vi "Begin.vi"(8 "error in":errorcluster) -> (0 "error out":errorcluster)   [LabVIEW 2014]
doc: "Called before other user functions, this VI is expected to open initial I/O refnums, load in file data, and do all program initialization. Notice that the <B>error out</B> terminal is simply used for data flow. Wiring it to other structures or subVIs ensures that this VI runs first."
uses:
  Robot/Forward Drive/Forward Drive Class/Forward Drive Config.ctl
  Robot/Motor with Encoders/Motors with Encoders Class/Motors with Encoders.lvclass
  Robot Actor Framework/Trace/Trace Controller Class/Config.ctl
  Robot/Motor with Encoders/Motors with Encoders Class/Motors with Encoders Config.ctl
  Comp Robot/Comp Motors with Encoders/Comp Motors with Encoders Class/Motor Controller Config.ctl
  Comp Robot/Comp Motors with Encoders/Comp Motors with Encoders Class/Encoder Config.ctl
  Robot/Driver/Driver Class/Driver Config.ctl
  Robot/Joystick/Joystick Class/Joystick.lvclass
  <vilib>/ActorFramework/Message Enqueuer/Message Enqueuer.lvclass
  Robot/Sideways Drive/Sideways Drive Class/Sideways Drive Config.ctl
  Comp Robot/Comp Xbox One Controller/Comp XBox One Controller Class/Comp X1 Config.ctl
  <vilib>/Rock Robotics/WPI/Joystick/WPI_JoystickDeviceEnum.ctl
  Dev Grabber/Dev Grabber Class/Dev Grabber Config.ctl
  <vilib>/Rock Robotics/WPI/Solenoid/WPI_SolenoidChannel.ctl
  Robot/Operator/Operator Class/Operator Config.ctl
  Robot/Elevator/Elevator Class/Elevator Config.ctl
  Comp Robot/Comp Motors with Brake/Comp Motors with Brake Class/Comp Motors with Brake Config.ctl
  <vilib>/Rock Robotics/WPI/DriverStation/WPI_DriverStationRobotMode2.ctl
  Comp Robot/Comp Pressure/Comp Pressure Class/Comp Pressure.lvclass
  Robot/Forward Drive/Forward Drive Class/Forward Drive.lvclass
  Robot/Sideways Drive/Sideways Drive Class/Sideways Drive.lvclass
  Comp Robot/Comp Trace Controller/Comp Trace Controller Class/Comp Trace Controller.lvclass
  Comp Robot/Comp Xbox One Controller/Comp XBox One Controller Class/Comp XBox One Controller.lvclass
  Robot/Driver/Driver Class/Driver.lvclass
  Robot/Operator/Operator Class/Operator.lvclass
  Robot/Joystick/Joystick Class/Config.ctl
  Comp Robot/Comp Motors with Encoders/Comp Motors with Encoders Class/Comp Motors with Encoders.lvclass
  Dev Grabber/Dev Grabber Class/Dev Grabber.lvclass
  Comp Robot/Comp Motors with Brake/Comp Motors with Brake Class/Comp Motors with Brake.lvclass
  Robot/Elevator/Elevator Class/Elevator.lvclass
  Robot/Joystick/Joystick Class/Joystick.lvclass/Joystick.ctl
  Comp Robot/Comp Xbox One Controller/Comp XBox One Controller Class/Comp XBox One Controller.lvclass/Comp XBox One Controller.ctl
  Robot Global Data.vi
  <vilib>/ActorFramework/Actor/Actor.lvclass
  Robot Actor Framework/Trace/Trace Controller Class/Trace Controller.lvclass
panel:
  in  "Configs":T1(tab)=enum."Sideways Motors "
  in  "Trace Controller Config":T2={"Folder Pattern"="/media/sd%s1", "Starting Letter Position"=1, "Min Free Space (MB)"=50.0, "Max Folders to Check"=10, "Trace Level"=enum."Informational"} {"Min Free Space (MB)" format="%#_13g"}
  in  "Left Motors Config":T3={"Counts  Per Revolution"=256, "Invert Encoder Direction"=FALSE, "Diameter of Revolution"=6.0, "Max RPM"=1500.0, "Encoder Control"=TRUE}
  in  "Left Master Motor Controller Config":T4={"Device Number"=9, "Invert Motor"=FALSE}
  in  "Left Slave Motor Controller Configs":T4[](array[typedef])=[{"Device Number"=10, "Invert Motor"=FALSE}]
  in  "Left Encoder Config":T5={"P"=1.0, "D"=0.0, "F"=0.01, "I"=0.01, "Reverse Feedback Sensor"=TRUE, "Encoder Codes Per Rev"=256}
  in  "Right Encoder Config 2":T3={"Counts  Per Revolution"=256, "Invert Encoder Direction"=FALSE, "Diameter of Revolution"=6.0, "Max RPM"=1500.0, "Encoder Control"=TRUE}
  in  "Right Master Motor Controller Config":T4={"Device Number"=4, "Invert Motor"=TRUE}
  in  "Right Slave Motor Controller Configs":T4[](array[typedef])=[{"Device Number"=5, "Invert Motor"=FALSE}]
  in  "Right Encoder Config":T5={"P"=1.0, "D"=0.0, "F"=0.01, "I"=0.01, "Reverse Feedback Sensor"=TRUE, "Encoder Codes Per Rev"=256}
  in  "Forward Drive Config":T6={"Left Motors with Encoders"=refnum, "Right Motors with Encoders"=refnum, "Encoder Control"=TRUE}
  in  "Driver Config":T7={"Joystick"=refnum, "Forward Drive"=refnum, "Sideways Drive"=refnum, "Percent Forward"=1.0, "Percent Sideways"=1.0}
  in  "Driver X1 Config":T8={"Joystick USB"=enum."USB 0", "Deadband"=0.1}
  in  "Sideways - Motors with Encoder Config":T3={"Counts  Per Revolution"=256, "Invert Encoder Direction"=FALSE, "Diameter of Revolution"=6.0, "Max RPM"=1500.0, "Encoder Control"=TRUE}
  in  "Sideways Drive Config":T10
  in  "Sideways Encoder Config":T5={"P"=1.0, "D"=0.0, "F"=0.01, "I"=0.01, "Reverse Feedback Sensor"=FALSE, "Encoder Codes Per Rev"=256}
  in  "Sideways Master Motor Controller Config":T4={"Device Number"=11, "Invert Motor"=TRUE}
  in  "Sideways Slave Motor Controller Configs":T4[](array[typedef])=[{"Device Number"=6, "Invert Motor"=FALSE}]
  in  "Operator XBox One Controller Config":T8={"Joystick USB"=enum."USB 1", "Deadband"=0.1}
  in  "Operator Config":T11
  in  "Dev Grabber Config":T12={"PCM CAN ID"=3, "Forward Solenoid Channel"=enum."Solenoid 0", "Reverse Solenoid Channel"=enum."Solenoid 1", "Left Motor CAN ID"=13, "Right Motor CAN ID"=8, "Left Motor Invert"=FALSE, "Right Motor Invert"=TRUE}
  in  "Elevator Config":T14
  in  "Elevator Master Motor Controller Config":T4={"Device Number"=7, "Invert Motor"=FALSE}
  in  "Ellevator  Motor Controller Configs":T4[](array[typedef])
  in  "Elevator Encoder Config":T5={"P"=1.0, "D"=0.0, "F"=0.01, "I"=0.01, "Reverse Feedback Sensor"=FALSE, "Encoder Codes Per Rev"=256}
  in  "Elevator Motors with Encoders Config":T3={"Counts  Per Revolution"=256, "Invert Encoder Direction"=FALSE, "Diameter of Revolution"=1.5, "Max RPM"=1000.0, "Encoder Control"=TRUE}
  in  "Comp Motors with Brake Config":T15={"Brake Channel"=enum."Solenoid 6", "Pneumatics CAN ID"=3}
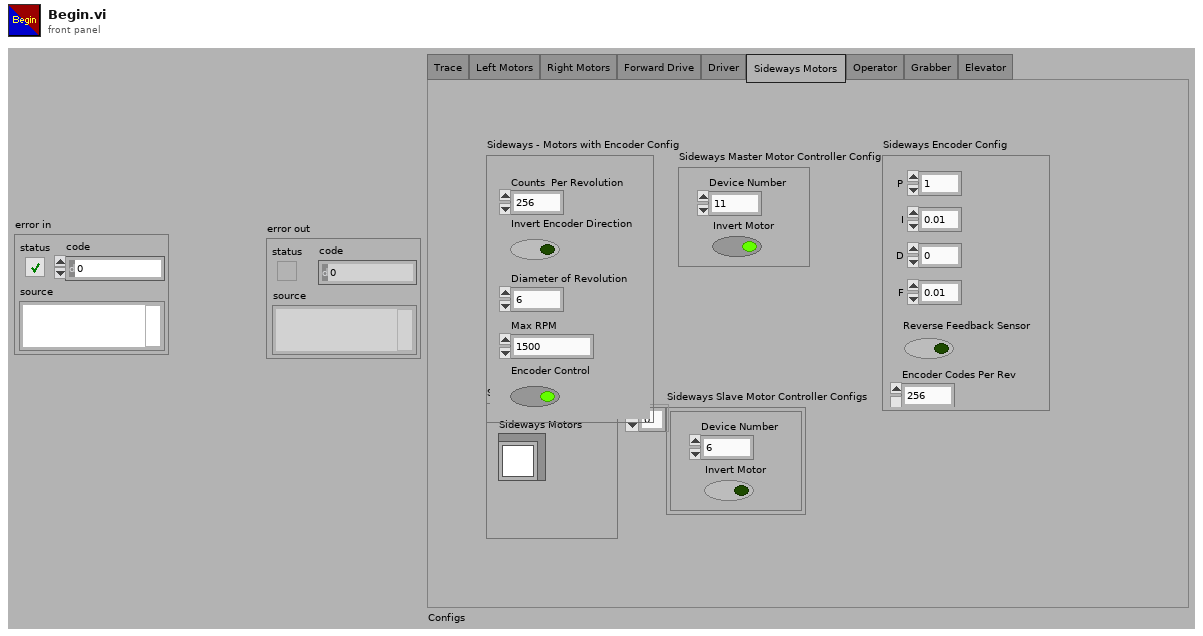
[diagram p1: front panel]
types:
  T1 = enum32{"Trace", "Left Motors", "Right Motors", "Forward Drive", "Driver", "Sideways Motors ", "Operator", "Grabber", "Elevator"}
  T2 = typedef "Robot Actor Framework.lvlib/Trace.lvlib/Trace Controller.lvclass/Config.ctl" = cluster{"Folder Pattern":string, "Starting Letter Position":i32, "Min Free Space (MB)":dbl, "Max Folders to Check":u32, "Trace Level":enum16{"Critical", "Error", "Warning", "Informational", "Debug"}}
  T3 = typedef "Motors with Encoders.lvlib/Motors with Encoders.lvclass/Motors with Encoders Config.ctl" = cluster{"Counts  Per Revolution":u32, "Invert Encoder Direction":bool, "Diameter of Revolution":dbl, "Max RPM":dbl, "Encoder Control":bool}
  T4 = typedef "Comp Motors with Encoders.lvlib/Comp Motors with Encoders.lvclass/Motor Controller Config.ctl" = cluster{"Device Number":u8, "Invert Motor":bool}
  T5 = typedef "Comp Motors with Encoders.lvlib/Comp Motors with Encoders.lvclass/Encoder Config.ctl" = cluster{"P":dbl, "D":dbl, "F":dbl, "I":dbl, "Reverse Feedback Sensor":bool, "Encoder Codes Per Rev":u16}
  T6 = typedef "Forward Drive.lvlib/Forward Drive.lvclass/Forward Drive Config.ctl" = cluster{"Left Motors with Encoders":refnum<class "Motors with Encoders.lvclass">, "Right Motors with Encoders":refnum<class "Motors with Encoders.lvclass">, "Encoder Control":bool}
  T7 = typedef "Driver.lvlib/Driver.lvclass/Driver Config.ctl" = cluster{"Joystick":refnum<class "Joystick.lvclass">, "Forward Drive":refnum<class "Message Enqueuer.lvclass">, "Sideways Drive":refnum<class "Message Enqueuer.lvclass">, "Percent Forward":dbl, "Percent Sideways":dbl}
  T8 = typedef "Comp XBox One Controller.lvlib/Comp XBox One Controller.lvclass/Comp X1 Config.ctl" = cluster{"Joystick USB":T9, "Deadband":dbl}
  T9 = typedef "WPI_JoystickDeviceEnum.ctl" = enum16{"USB 0", "USB 1", "USB 2", "USB 3", "USB 4", "USB 5"}
  T10 = typedef "Sideways Drive.lvlib/Sideways Drive.lvclass/Sideways Drive Config.ctl" = cluster{"Sideways Motors":refnum<class "Motors with Encoders.lvclass">}
  T11 = typedef "Operator.lvlib/Operator.lvclass/Operator Config.ctl" = cluster{"Grabber":refnum<class "Message Enqueuer.lvclass">, "Joystick Class":refnum<class "Joystick.lvclass">, "Elevator":refnum<class "Message Enqueuer.lvclass">}
  T12 = typedef "Dev Grabber.lvlib/Dev Grabber.lvclass/Dev Grabber Config.ctl" = cluster{"PCM CAN ID":u8, "Forward Solenoid Channel":T13, "Reverse Solenoid Channel":T13, "Left Motor CAN ID":u8, "Right Motor CAN ID":u8, "Left Motor Invert":bool, "Right Motor Invert":bool}
  T13 = typedef "WPI_SolenoidChannel.ctl" = enum8{"Solenoid 0", "Solenoid 1", "Solenoid 2", "Solenoid 3", "Solenoid 4", "Solenoid 5", "Solenoid 6", "Solenoid 7", "Invalid"}
  T14 = typedef "Elevator.lvlib/Elevator.lvclass/Elevator Config.ctl" = cluster{"Motors with Encoders ":refnum<class "Motors with Encoders.lvclass">}
  T15 = typedef "Comp Motors with Brake.lvlib/Comp Motors with Brake.lvclass/Comp Motors with Brake Config.ctl" = cluster{"Brake Channel":T13, "Pneumatics CAN ID":u8}
  T16 = enum16{"Critical", "Error", "Warning", "Informational", "Debug"}
  T17 = typedef "Joystick.lvlib/Joystick.lvclass/Config.ctl" = cluster{"Thumbstick Deadband":dbl}
  T18 = typedef "WPI_DriverStationRobotMode2.ctl" = enum16{"Autonomous Disabled", "Autonomous Enabled", "Teleop Disabled", "Teleop Enabled", "Disconnected", "Finish", "Test Disabled", "Test Enabled", "Emergency Stopped"}
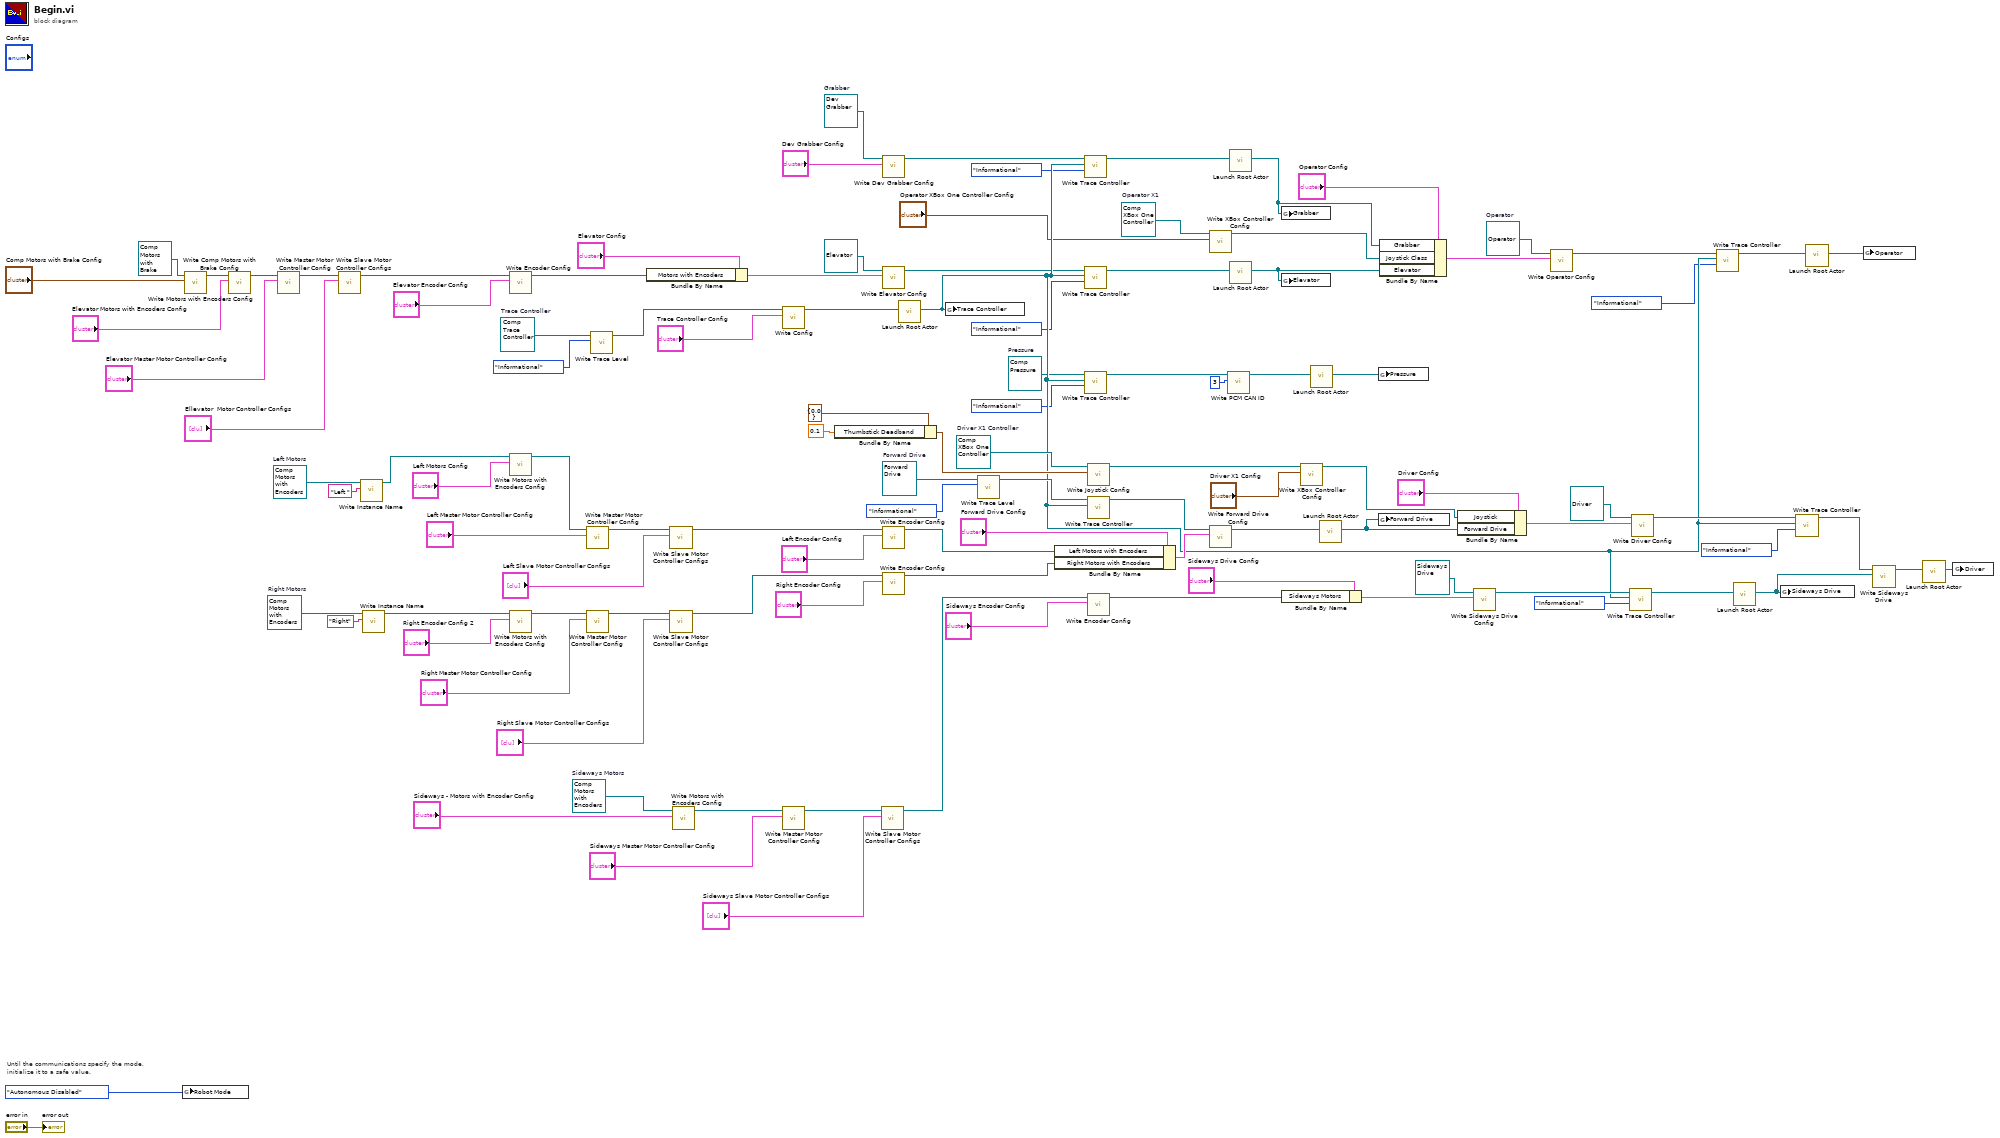
[diagram p0: block diagram]
diagram:
  w35 = refnum<class "Dev Grabber.lvclass"> refnum  # Grabber
  w51 = refnum<class "Comp Motors with Encoders.lvclass"> refnum  # Sideways Motors
  w70 = refnum<class "Comp Motors with Encoders.lvclass"> refnum  # Right Motors
  w83 = refnum<class "Comp Motors with Encoders.lvclass"> refnum  # Left Motors
  w19 = refnum<class "Comp XBox One Controller.lvclass"> refnum  # Operator X1
  w29 = refnum<class "Operator.lvclass"> refnum  # Operator
  w91 = refnum<class "Comp XBox One Controller.lvclass"> refnum  # Driver X1 Controller
  w96 = refnum<class "Comp Trace Controller.lvclass"> refnum  # Trace Controller
  w102 = refnum<class "Forward Drive.lvclass"> refnum  # Forward Drive
  w6 = refnum<class "Comp Pressure.lvclass"> refnum  # Pressure
  # "Until the communications specify the mode,\ninitialize it to a safe value."
  n1 = global write "Robot Global Data.vi" "Robot Mode"(WPI_DriverStationRobotMode2."Autonomous Disabled" ("Robot Mode")) -> ()
  n2 = call-dynamic "Write Comp Motors with Brake Config.vi"("Comp Motors with Brake Config"="Comp Motors with Brake Config", "Comp Motors with Brake in"=refnum<class "Comp Motors with Brake.lvclass"> refnum ("Comp Motors with Brake.lvlib:Comp Motors with Brake.lvclass")) -> ("Comp Motors with Brake out"=w3:refnum<class "Comp Motors with Brake.lvclass">)  [unwired: 8 in, 1 out]
  n3 = call-dynamic "Write Motors with Encoders Config.vi"("Motors with Encoders Config"="Elevator Motors with Encoders Config", "Motors with Encoders in"=w3) -> ("Motors with Encoders out"=w9:refnum<class "Comp Motors with Brake.lvclass">)  [unwired: 8 in, 1 out]
  n4 = call-dynamic "Write Master Motor Controller Config.vi"("Master Motor Controller Config"="Elevator Master Motor Controller Config", "Comp Motors with Encoders in"=w9) -> ("Comp Motors with Encoders out"=w94:refnum<class "Comp Motors with Brake.lvclass">)  [unwired: 8 in, 1 out]
  n5 = call-dynamic "Write Slave Motor Controller Configs.vi"("Slave Motor Controller Configs"="Ellevator  Motor Controller Configs", "Comp Motors with Encoders in"=w94) -> ("Comp Motors with Encoders out"=w12:refnum<class "Comp Motors with Brake.lvclass">)  [unwired: 8 in, 1 out]
  n6 = call-dynamic "Write Instance Name.vi"("Instance Name"="Left ", "System Actor in"=w83) -> ("System Actor out"=w81:refnum<class "Comp Motors with Encoders.lvclass">)  [unwired: 8 in, 1 out]
  n7 = call-dynamic "Write Instance Name.vi"("Instance Name"="Right", "System Actor in"=w70) -> ("System Actor out"=w68:refnum<class "Comp Motors with Encoders.lvclass">)  [unwired: 8 in, 1 out]
  n8 = call-dynamic "Write Encoder Config.vi"("Encoder Config"="Elevator Encoder Config", "Comp Motors with Encoders in"=w12) -> ("Comp Motors with Encoders out"=w11:refnum<class "Comp Motors with Brake.lvclass">)  [unwired: 8 in, 1 out]
  n9 = call-dynamic "Write Motors with Encoders Config.vi"("Motors with Encoders Config"="Left Motors Config", "Motors with Encoders in"=w81) -> ("Motors with Encoders out"=w80:refnum<class "Comp Motors with Encoders.lvclass">)  [unwired: 8 in, 1 out]
  n10 = call-dynamic "Write Motors with Encoders Config.vi"("Motors with Encoders Config"="Right Encoder Config 2", "Motors with Encoders in"=w68) -> ("Motors with Encoders out"=w67:refnum<class "Comp Motors with Encoders.lvclass">)  [unwired: 8 in, 1 out]
  n11 = call-dynamic "Write Master Motor Controller Config.vi"("Master Motor Controller Config"="Left Master Motor Controller Config", "Comp Motors with Encoders in"=w80) -> ("Comp Motors with Encoders out"=w79:refnum<class "Comp Motors with Encoders.lvclass">)  [unwired: 8 in, 1 out]
  n12 = call-dynamic "Write Master Motor Controller Config.vi"("Master Motor Controller Config"="Right Master Motor Controller Config", "Comp Motors with Encoders in"=w67) -> ("Comp Motors with Encoders out"=w66:refnum<class "Comp Motors with Encoders.lvclass">)  [unwired: 8 in, 1 out]
  n13 = call-dynamic "Write Trace Level.vi"("Trace Level"=T16."Informational", "System Actor in"=w96) -> ("System Actor out"=w93:refnum<class "Comp Trace Controller.lvclass">)  [unwired: 8 in, 1 out]
  n14 = Bundle By Name(cluster="Elevator Config", "Motors with Encoders"=w11) -> (w16:T14)
  n15 = call-dynamic "Write Slave Motor Controller Configs.vi"("Slave Motor Controller Configs"="Left Slave Motor Controller Configs", "Comp Motors with Encoders in"=w79) -> ("Comp Motors with Encoders out"=w78:refnum<class "Comp Motors with Encoders.lvclass">)  [unwired: 8 in, 1 out]
  n16 = call-dynamic "Write Slave Motor Controller Configs.vi"("Slave Motor Controller Configs"="Right Slave Motor Controller Configs", "Comp Motors with Encoders in"=w66) -> ("Comp Motors with Encoders out"=w65:refnum<class "Comp Motors with Encoders.lvclass">)  [unwired: 8 in, 1 out]
  n17 = call-dynamic "Write Motors with Encoders Config.vi"("Motors with Encoders Config"="Sideways - Motors with Encoder Config", "Motors with Encoders in"=w51) -> ("Motors with Encoders out"=w50:refnum<class "Comp Motors with Encoders.lvclass">)  [unwired: 8 in, 1 out]
  n18 = call-dynamic "Write Config.vi"("Config"="Trace Controller Config", "Trace Controller in"=w93) -> ("Trace Controller out"=w92:refnum<class "Comp Trace Controller.lvclass">)  [unwired: 8 in, 1 out]
  n19 = call-dynamic "Write Master Motor Controller Config.vi"("Master Motor Controller Config"="Sideways Master Motor Controller Config", "Comp Motors with Encoders in"=w50) -> ("Comp Motors with Encoders out"=w49:refnum<class "Comp Motors with Encoders.lvclass">)  [unwired: 8 in, 1 out]
  n20 = Bundle By Name(cluster=T17 {"Thumbstick Deadband"=0.0} ("Config"), "Thumbstick Deadband"=0.1) -> (w88:T17)
  n21 = call-dynamic "Write Slave Motor Controller Configs.vi"("Slave Motor Controller Configs"="Sideways Slave Motor Controller Configs", "Comp Motors with Encoders in"=w49) -> ("Comp Motors with Encoders out"=w48:refnum<class "Comp Motors with Encoders.lvclass">)  [unwired: 8 in, 1 out]
  n22 = call-dynamic "Write Dev Grabber Config.vi"("Dev Grabber Config"="Dev Grabber Config", "Dev Grabber in"=w35) -> ("Dev Grabber out"=w34:refnum<class "Dev Grabber.lvclass">)  [unwired: 8 in, 1 out]
  n23 = call-dynamic "Write Elevator Config.vi"("Elevator Config"=w16, "Elevator in"=refnum<class "Elevator.lvclass"> refnum ("Elevator.lvlib:Elevator.lvclass")) -> ("Elevator out"=w1:refnum<class "Elevator.lvclass">)  [unwired: 8 in, 1 out]
  n24 = call-dynamic "Write Encoder Config.vi"("Encoder Config"="Left Encoder Config", "Comp Motors with Encoders in"=w78) -> ("Comp Motors with Encoders out"=w72:refnum<class "Comp Motors with Encoders.lvclass">)  [unwired: 8 in, 1 out]
  n25 = call-dynamic "Write Encoder Config.vi"("Encoder Config"="Right Encoder Config", "Comp Motors with Encoders in"=w65) -> ("Comp Motors with Encoders out"=w64:refnum<class "Comp Motors with Encoders.lvclass">)  [unwired: 8 in, 1 out]
  n26 = call <vilib>:"Launch Root Actor.vi"("Actor"=w92) -> ("Actor's Enqueuer"=w33:refnum<class "Message Enqueuer.lvclass">)  [unwired: 9 in, 1 out]
  n27 = global write "Robot Global Data.vi" "Trace Controller"(w33) -> ()
  n28 = call-dynamic "Write Trace Level.vi"("Trace Level"=T16."Informational", "System Actor in"=w102) -> ("System Actor out"=w100:refnum<class "Forward Drive.lvclass">)  [unwired: 8 in, 1 out]
  n29 = Bundle By Name(cluster="Forward Drive Config", "Left Motors with Encoders"=w72, "Right Motors with Encoders"=w64) -> (w73:T6)
  n30 = call-dynamic "Write Trace Controller.vi"("Trace Level"=T16."Informational", "Trace Controller"=w33, "System Actor in"=w34) -> ("System Actor out"=w30:refnum<class "Dev Grabber.lvclass">)  [unwired: 7 in, 1 out]
  n31 = call-dynamic "Write Trace Controller.vi"("Trace Level"=T16."Informational", "Trace Controller"=w33, "System Actor in"=w1) -> ("System Actor out"=w15:refnum<class "Elevator.lvclass">)  [unwired: 7 in, 1 out]
  n32 = call-dynamic "Write Trace Controller.vi"("Trace Level"=T16."Informational", "Trace Controller"=w33, "System Actor in"=w6) -> ("System Actor out"=w105:refnum<class "Comp Pressure.lvclass">)  [unwired: 7 in, 1 out]
  n33 = call "Write Joystick Config.vi"("Config"=w88, "Joystick in"=w91) -> ("Joystick out"=w90:refnum<class "Comp XBox One Controller.lvclass">)  [unwired: 8 in, 1 out]
  n34 = call-dynamic "Write Trace Controller.vi"("Trace Controller"=w33, "System Actor in"=w100) -> ("System Actor out"=w86:refnum<class "Forward Drive.lvclass">)  [unwired: 8 in, 1 out]
  n35 = call-dynamic "Write Encoder Config.vi"("Encoder Config"="Sideways Encoder Config", "Comp Motors with Encoders in"=w48) -> ("Comp Motors with Encoders out"=w42:refnum<class "Comp Motors with Encoders.lvclass">)  [unwired: 8 in, 1 out]
  n36 = call "Write XBox Controller Config.vi"("XBox One Controller Config"="Operator XBox One Controller Config", "Comp XBox One Controller in"=w19) -> ("Comp XBox One Controller out"=w24:refnum<class "Comp XBox One Controller.lvclass">)  [unwired: 8 in, 1 out]
  n37 = call-dynamic "Write Forward Drive Config.vi"("Forward Drive Config"=w73, "Forward Drive in"=w86) -> ("Forward Drive out"=w71:refnum<class "Forward Drive.lvclass">)  [unwired: 8 in, 1 out]
  n38 = call-dynamic "Write PCM CAN ID.vi"("PCM CAN ID"=u8 3, "Comp Pressure in"=w105) -> ("Comp Pressure out"=w104:refnum<class "Comp Pressure.lvclass">)  [unwired: 8 in, 1 out]
  n39 = call <vilib>:"Launch Root Actor.vi"("Actor"=w30) -> ("Actor's Enqueuer"=w21:refnum<class "Message Enqueuer.lvclass">)  [unwired: 9 in, 1 out]
  n40 = call <vilib>:"Launch Root Actor.vi"("Actor"=w15) -> ("Actor's Enqueuer"=w23:refnum<class "Message Enqueuer.lvclass">)  [unwired: 9 in, 1 out]
  n41 = global write "Robot Global Data.vi" "Grabber"(w21) -> ()
  n42 = global write "Robot Global Data.vi" "Elevator"(w23) -> ()
  n43 = Bundle By Name(cluster="Sideways Drive Config", "Sideways Motors"=w42) -> (w43:T10)
  n44 = call "Write XBox Controller Config.vi"("XBox One Controller Config"="Driver X1 Config", "Comp XBox One Controller in"=w90) -> ("Comp XBox One Controller out"=w55:refnum<class "Comp XBox One Controller.lvclass">)  [unwired: 8 in, 1 out]
  n45 = call <vilib>:"Launch Root Actor.vi"("Actor"=w104) -> ("Actor's Enqueuer"=w107:refnum<class "Message Enqueuer.lvclass">)  [unwired: 9 in, 1 out]
  n46 = call <vilib>:"Launch Root Actor.vi"("Actor"=w71) -> ("Actor's Enqueuer"=w53:refnum<class "Message Enqueuer.lvclass">)  [unwired: 9 in, 1 out]
  n47 = global write "Robot Global Data.vi" "Pressure"(w107) -> ()
  n48 = global write "Robot Global Data.vi" "Forward Drive"(w53) -> ()
  n49 = Bundle By Name(cluster="Operator Config", "Grabber"=w21, "Joystick Class"=w24, "Elevator"=w23) -> (w25:T11)
  n50 = Bundle By Name(cluster="Driver Config", "Joystick"=w55, "Forward Drive"=w53) -> (w56:T7)
  n51 = call-dynamic "Write Sideways Drive Config.vi"("Sideways Drive Config"=w43, "Sideways Drive in"=refnum<class "Sideways Drive.lvclass"> refnum ("Sideways Drive.lvlib:Sideways Drive.lvclass")) -> ("Sideways Drive out"=w45:refnum<class "Sideways Drive.lvclass">)  [unwired: 8 in, 1 out]
  n52 = call-dynamic "Write Operator Config.vi"("Operator Config"=w25, "Operator in"=w29) -> ("Operator out"=w28:refnum<class "Operator.lvclass">)  [unwired: 8 in, 1 out]
  n53 = call-dynamic "Write Trace Controller.vi"("Trace Level"=T16."Informational", "Trace Controller"=w33, "System Actor in"=w45) -> ("System Actor out"=w41:refnum<class "Sideways Drive.lvclass">)  [unwired: 7 in, 1 out]
  n54 = call-dynamic "Write Driver Config.vi"("Driver Config"=w56, "Driver in"=refnum<class "Driver.lvclass"> refnum ("Driver.lvlib:Driver.lvclass")) -> ("Driver out"=w59:refnum<class "Driver.lvclass">)  [unwired: 8 in, 1 out]
  n55 = call-dynamic "Write Trace Controller.vi"("Trace Level"=T16."Informational" ("Operatlor Trace Level"), "Trace Controller"=w33, "System Actor in"=w28) -> ("System Actor out"=w22:refnum<class "Operator.lvclass">)  [unwired: 7 in, 1 out]
  n56 = call <vilib>:"Launch Root Actor.vi"("Actor"=w41) -> ("Actor's Enqueuer"=w97:refnum<class "Message Enqueuer.lvclass">)  [unwired: 9 in, 1 out]
  n57 = global write "Robot Global Data.vi" "Sideways Drive"(w97) -> ()
  n58 = call-dynamic "Write Trace Controller.vi"("Trace Level"=T16."Informational", "Trace Controller"=w33, "System Actor in"=w59) -> ("System Actor out"=w52:refnum<class "Driver.lvclass">)  [unwired: 7 in, 1 out]
  n59 = call <vilib>:"Launch Root Actor.vi"("Actor"=w22) -> ("Actor's Enqueuer"=w95:refnum<class "Message Enqueuer.lvclass">)  [unwired: 9 in, 1 out]
  n60 = global write "Robot Global Data.vi" "Operator"(w95) -> ()
  n61 = call-dynamic "Write Sideways Drive.vi"("Actor Framework:Message Enqueuer"=w97, "Driver in"=w52) -> ("Driver out"=w98:refnum<class "Driver.lvclass">)  [unwired: 8 in, 1 out]
  n62 = call <vilib>:"Launch Root Actor.vi"("Actor"=w98) -> ("Actor's Enqueuer"=w99:refnum<class "Message Enqueuer.lvclass">)  [unwired: 9 in, 1 out]
  n63 = global write "Robot Global Data.vi" "Driver"(w99) -> ()
  "error out" <- "error in"
